vi "values checker.vi"(8 "error in (no error)":errorcluster, 9 "values":string[](array[string]), 10 "values 2":string[](array[string]), 11 "sectors":string[][](array[string])) -> (0 "error out":errorcluster)   [LabVIEW 2024]
uses:
  <vilib>/Utility/error.llb/Error Cluster From Error Code.vi
  <vilib>/ErrorRing/Error Ring.xnode
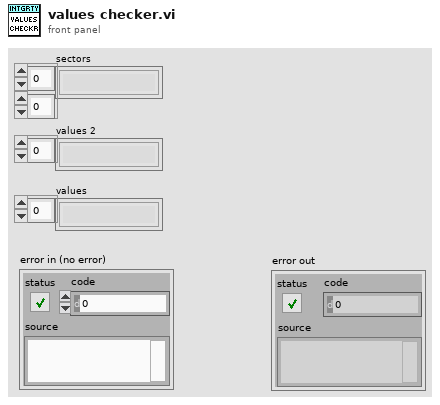
[diagram p1: front panel]
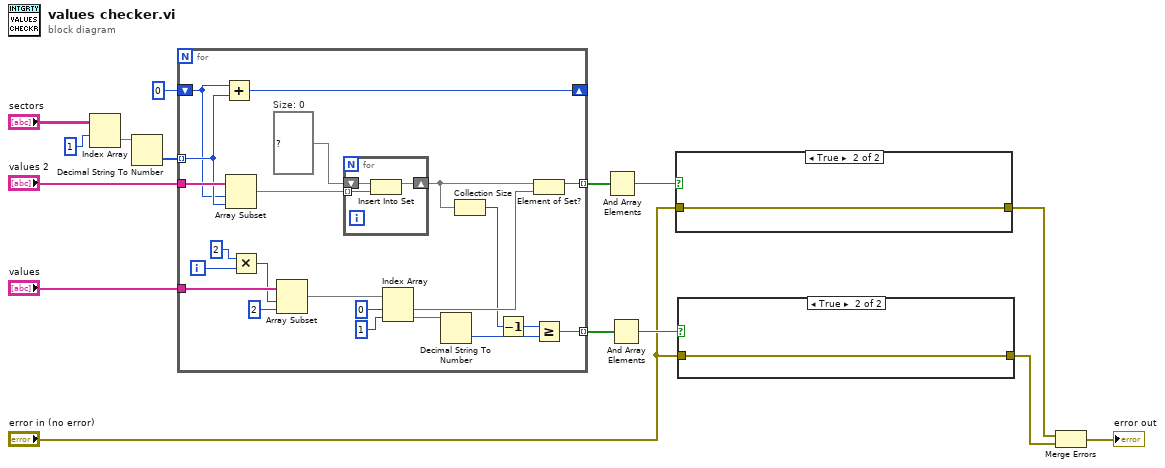
[diagram p0: block diagram]
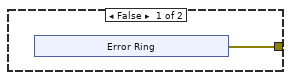
[diagram p2: hidden frame]
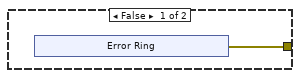
[diagram p3: hidden frame]
diagram:
  n1 = Index Array(array="sectors", index (row)=1) -> (element=w11:string[])  [unwired: 1 in]
  n2 = Decimal String To Number(string=w11) -> (number=w14:i32[])  [unwired: 2 in, 1 out]
  n3 = for {
    tunnel: w14 -> [w34] mode=indexing
    shift-right: [w37] -> _
    shift-left: 0 -> [w33]
    tunnel: "values 2" -> [w36]
    tunnel: "values" -> [w35]
    tunnel: [w18] -> w8 mode=indexing
    tunnel: [w17] -> w7 mode=indexing
    i -> [w31]
    w27 = set{string} {}  # Size: 0
    n4 = Add(x=w33, y=w34) -> (x+y=w37:i32)
    n5 = Array Subset(array=w36, index=w33, length=w34) -> (w28:string[])
    n6 = Multiply(x=2, y=w31) -> (x*y=w29:i32)
    n7 = Array Subset(array=w35, index=w29, length=2) -> (w26:string[])
    n8 = for {
      tunnel: w28 -> [w40] mode=indexing
      shift-right: [w38] -> w23
      shift-left: w27 -> [w39]
      n9 = Insert Into Set(10:w40, 11:w39) -> (3:w38:set{string})  [unwired: 1 out]
    }
    n10 = Index Array(array=w26, index #1=0 ("index"), index #2=1 ("index")) -> (element #1=w22:string, element #2=w21:string)
    n11 = Decimal String To Number(string=w21) -> (number=w19:i32)  [unwired: 2 in, 1 out]
    n12 = Collection Size(1:w23) -> (0:w20:i32)
    n13 = Decrement(x=w20) -> (x-1=w16:i32)
    n14 = Element of Set?(10:w22, 11:w23) -> (3:w18:bool)
    n15 = Greater Or Equal?(x=w16, y=w19) -> (x >= y?=w17:bool)
  }
  n16 = And Array Elements(Boolean array=w8) -> (logical AND=w5:bool)
  n17 = And Array Elements(Boolean array=w7) -> (logical AND=w6:bool)
  n18 = case shown="True" w5 {
    tunnel: [w41 w47] -> w1
    tunnel: "error in (no error)" -> [_ w47]
    frame False {
      n19 = xnode ("Error Ring")() -> ("error out"=w41:errorcluster)
    }
    frame True {
    }
  }
  n20 = case shown="True" w6 {
    tunnel: [w48 w54] -> w2
    tunnel: "error in (no error)" -> [_ w54]
    frame False {
      n21 = xnode ("Error Ring")() -> ("error out"=w48:errorcluster)
    }
    frame True {
    }
  }
  n22 = Merge Errors(w1, w2) -> (→"error out":errorcluster)
